vi "Trajectory_SampleReverseTEST_ORIENT.vi"(9 "Time":dbl, 11 "InputTRAJECTORY":T5 {"States"."POSE"."ROTATION"."SIN" format="%13.4f"; "States"."POSE"."ROTATION"."COS" format="%13.4f"; "States"."POSE"."ROTATION"."VALUE" format="%13.4f"; "States"."POSE"."TRANSLATION"."Y" format="%14.3f"; "States"."POSE"."TRANSLATION"."X" format="%14.3f"; "TotalTImeSecs" format="%20.3f"}) -> (3 "OutputTRAJ_STATE":T1={"TimeSeconds"=0.0, "Velocity"=0.0, "Acceleration"=0.0, "POSE"={"TRANSLATION"={"X"=0.0, "Y"=0.0}, "ROTATION"={"VALUE"=0.0, "COS"=1.0, "SIN"=0.0}}, "Curvature"=0.0} {"POSE"."ROTATION"."SIN" format="%13.4f"; "POSE"."ROTATION"."COS" format="%13.4f"; "POSE"."ROTATION"."VALUE" format="%13.4f"; "POSE"."TRANSLATION"."Y" format="%14.3f"; "POSE"."TRANSLATION"."X" format="%14.3f"})   [LabVIEW 2019]
doc: "Sample the trajectory at a point in time. The trajectory is sampled in reverse such that the ending time becomes 0 and the beginning time is the maximum time. The selected trajectory state is then transformed to be relative to end of the trajectory.\n\nThis routine does not exist in WPILIB\n \nParameters:\n - InputTrajectory - The Trajectory data structure\n - time - The point in time since the beginning of the trajectory to sample. (seconds)\n\nReturns:\n - OutputTrajState - The state at that point in time."
uses:
  <vilib>/Rock Robotics/WPI/ThirdParty/JAS_Junk/TrajLib/Translation_Create.vi
  <vilib>/Rock Robotics/WPI/ThirdParty/JAS_Junk/TrajLib/Rotation_UnaryMinus.vi
  <vilib>/Rock Robotics/WPI/ThirdParty/JAS_Junk/TrajLib/Translation_RotateBy.vi
  <vilib>/Rock Robotics/WPI/ThirdParty/JAS_Junk/TrajLib/Translation_Minus.vi
  <vilib>/Rock Robotics/WPI/ThirdParty/JAS_Junk/TrajLib/Rotation_Minus.vi
  <vilib>/Rock Robotics/WPI/ThirdParty/JAS_Junk/TrajLib/Translation_Plus.vi
  <vilib>/Rock Robotics/WPI/ThirdParty/JAS_Junk/TrajLib/Rotation_Plus.vi
  <vilib>/Rock Robotics/WPI/ThirdParty/JAS_Junk/TrajLib/Pose_New_TRRO.vi
  <vilib>/Rock Robotics/WPI/ThirdParty/JAS_Junk/TrajLib/Rotation_RotateBy.vi
  <vilib>/Rock Robotics/WPI/ThirdParty/JAS_Junk/TrajLib/Rotation_CreateXY.vi
  <vilib>/Rock Robotics/WPI/ThirdParty/JAS_Junk/TrajLib/Util_CalcDist.vi
  <vilib>/Rock Robotics/WPI/ThirdParty/JAS_Junk/TrajLib/Trajectory_Library.lvlib
  <vilib>/Rock Robotics/WPI/ThirdParty/JAS_Junk/TrajLib/TRANSLATION2D.ctl
  <vilib>/Rock Robotics/WPI/ThirdParty/JAS_Junk/TrajLib/ROTATION2D.ctl
  <vilib>/Rock Robotics/WPI/ThirdParty/JAS_Junk/TrajLib/POSE2D.ctl
  <vilib>/Rock Robotics/WPI/ThirdParty/JAS_Junk/TrajLib/TRAJ_STATE.ctl
  <vilib>/Rock Robotics/WPI/ThirdParty/JAS_Junk/TrajLib/TRAJECTORY.ctl
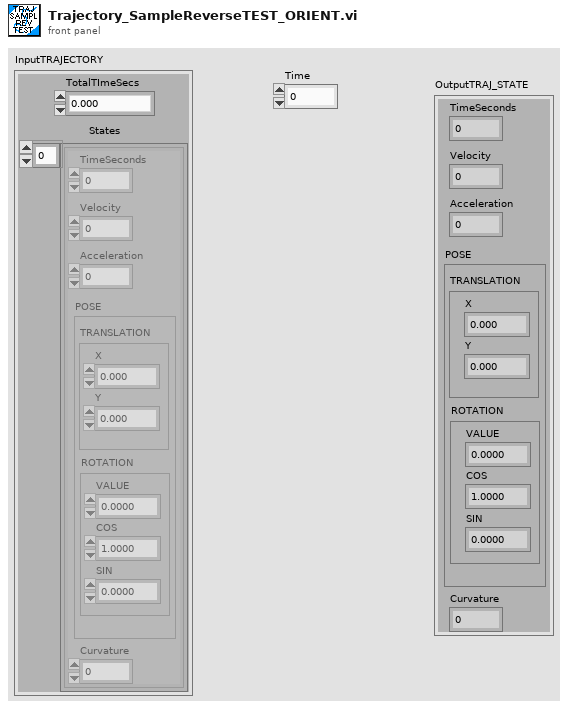
[diagram p1: front panel]
types:
  T1 = typedef "Trajectory_Library.lvlib/TRAJ_STATE.ctl" = cluster{"TimeSeconds":dbl, "Velocity":dbl, "Acceleration":dbl, "POSE":T2, "Curvature":dbl}
  T2 = typedef "Trajectory_Library.lvlib/POSE2D.ctl" = cluster{"TRANSLATION":T3, "ROTATION":T4}
  T3 = typedef "Trajectory_Library.lvlib/TRANSLATION2D.ctl" = cluster{"X":dbl, "Y":dbl}
  T4 = typedef "Trajectory_Library.lvlib/ROTATION2D.ctl" = cluster{"VALUE":dbl, "COS":dbl, "SIN":dbl}
  T5 = typedef "Trajectory_Library.lvlib/TRAJECTORY.ctl" = cluster{"TotalTImeSecs":dbl, "States":T1[]}
  T6 = typedef "Trajectory_Library.lvlib/TRANSFORM2D.ctl" = cluster{"TRANSLATION":T3, "ROTATION":T4}
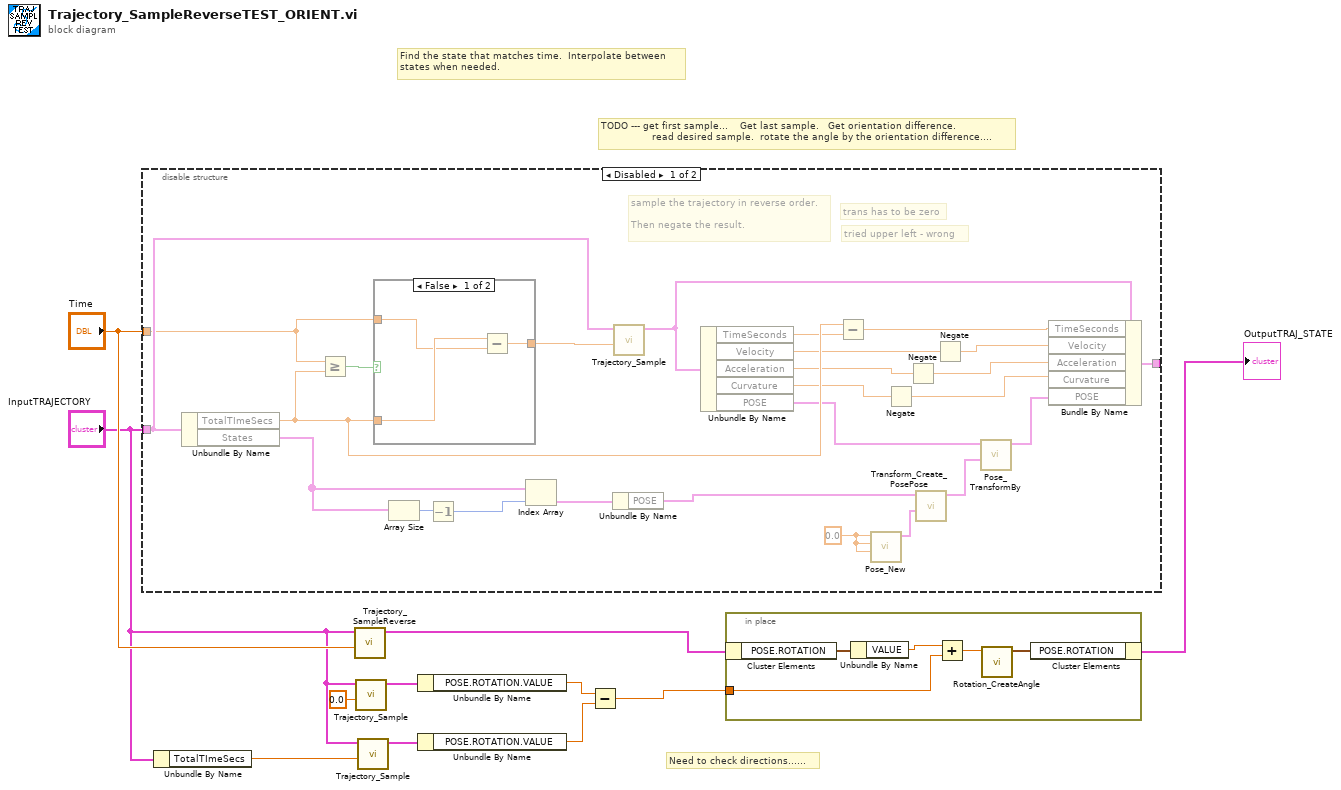
[diagram p0: block diagram]
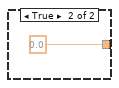
[diagram p2: hidden frame]
diagram:
  # "Need to check directions......"
  # "TODO --- get first sample...    Get last sample.   Get orientation difference.\n                 read desired sample.  rotate the angle by the orientation difference...."
  # "Find the state that matches time.  Interpolate between\nstates when needed."
  n1 = disable-structure shown="Disabled" {
    disable-tunnel: "InputTRAJECTORY" -> [w35 _]
    disable-tunnel: "Time" -> [w19 _]
    disable-tunnel: [w17 _] -> _
    frame Disabled {
      w13 = 0.0 ("X")
      # "tried upper left - wrong"
      # "trans has to be zero"
      # "sample the trajectory in reverse order.\n\nThen negate the result."
      n2 = Unbundle By Name(w35) -> ("TotalTImeSecs"=w30:dbl, "States"=w32:T1[])
      n3 = Greater Or Equal?(x=w19, y=w30) -> (x >= y?=w36:bool)
      n4 = case shown="False" w36 {
        tunnel: [w37 0.0] -> w18
        tunnel: w30 -> [w39 _]
        tunnel: w19 -> [w38 _]
        frame False {
          n5 = Subtract(x=w39, y=w38) -> (x-y=w37:dbl)
        }
        frame True {
        }
      }
      n6 = Array Size(array=w32) -> (size(s)=w34:i32)
      n7 = Decrement(x=w34) -> (x-1=w33:i32)
      n8 = Index Array(array=w32, index=w33) -> (element=w21:T1)
      n9 = Unbundle By Name(w21) -> ("POSE"=w14:T2)
      n10 = call <vilib>:"Trajectory_Sample.vi"("Time"=w18, "InputTRAJECTORY"=w35) -> ("OutputTRAJ_STATE"=w31:T1)  [unwired: 9 in]
      n11 = Unbundle By Name(w31) -> ("TimeSeconds"=w29:dbl, "Velocity"=w27:dbl, "Acceleration"=w25:dbl, "Curvature"=w24:dbl, "POSE"=w16:T2)
      n12 = Subtract(x=w30, y=w29) -> (x-y=w28:dbl)
      n13 = call <vilib>:"Pose_New.vi"("Heading"=w13, "Y"=w13, "X"=w13) -> ("out POSe"=w12:T2)  [unwired: 8 in]
      n14 = Negate(x=w24) -> (-x=w22:dbl)
      n15 = Negate(x=w25) -> (-x=w23:dbl)
      n16 = call <vilib>:"Transform_Create_PosePose.vi"("last POSE"=w12, "initial POSE"=w14) -> ("TRANSFORM"=w20:T6)  [unwired: 9 in]
      n17 = Negate(x=w27) -> (-x=w26:dbl)
      n18 = call <vilib>:"Pose_TransformBy.vi"("other TRANSFORM"=w20, "in POSE"=w16) -> ("out POSE"=w15:T2)  [unwired: 9 in]
      n19 = Bundle By Name(cluster=w31, "TimeSeconds"=w28, "Velocity"=w26, "Acceleration"=w23, "Curvature"=w22, "POSE"=w15) -> (w17:T1)
    }
    frame Enabled {
    }
  }
  n20 = Unbundle By Name("InputTRAJECTORY") -> ("TotalTImeSecs"=w8:dbl)
  n21 = call <vilib>:"Trajectory_SampleReverse.vi"("Time"="Time", "InputTRAJECTORY"="InputTRAJECTORY") -> ("OutputTRAJ_STATE"=w3:T1)  [unwired: 9 in]
  n22 = call <vilib>:"Trajectory_Sample.vi"("Time"=0.0, "InputTRAJECTORY"="InputTRAJECTORY") -> ("OutputTRAJ_STATE"=w6:T1)  [unwired: 9 in]
  n23 = call <vilib>:"Trajectory_Sample.vi"("Time"=w8, "InputTRAJECTORY"="InputTRAJECTORY") -> ("OutputTRAJ_STATE"=w7:T1)  [unwired: 9 in]
  n24 = Unbundle By Name(w6) -> ("POSE.ROTATION.VALUE"=w5:dbl)
  n25 = Unbundle By Name(w7) -> ("POSE.ROTATION.VALUE"=w4:dbl)
  n26 = Subtract(x=w5, y=w4) -> (x-y=w2:dbl)
  n27 = in-place {
    in-place-border: w2 -> [w41]
    n28 = in-place-cluster #1(w3) -> ("POSE.ROTATION"=w45:T4)
    n29 = Unbundle By Name(w45) -> ("VALUE"=w44:dbl)
    n30 = Add(x=w44, y=w41) -> (x+y=w43:dbl)
    n31 = call <vilib>:"Rotation_CreateAngle.vi"("Angle"=w43) -> ("ROTATION"=w42:T4)  [unwired: 10 in]
    n32 = in-place-cluster #1("POSE.ROTATION"=w42) -> (→"OutputTRAJ_STATE":T1)
  }
